vi "SECoP_dataGetAdditionalIndex.vi"(7 "Position":u32, 8 "error in (no error)":errorcluster, 9 "key name":string, 10 "SECoP_dataPtr":T1 {"ptr64" format="%.0x"; "ptr32" format="%.0x"}, 11 "DLL path (in)":T2) -> (0 "error out":errorcluster, 2 "Index":u32, 3 "DLL path (out)":T2)   [LabVIEW 2023, in "SECoP.lvlib"]
doc: "Call <b>\"SECoP_dataGetAdditionalIndex.vi\"</b> to find the index of named additional item of SECoP_dataPtr.\n\n<b>DLL path</b> input and output of cluster from \"SECoP-Initialize.vi\"\n<b>SECoP_dataPtr</b> data to access\n<b>Position</b> points to a virtual flattened entry of the data type\n<b>key name</b> name of the requested additional item of SECoP_dataPtr\n<b>Index</b> index of additional item (or 0xFFFFFFFF if not found)"
uses:
  SECoP.lvlib
  SECoP-libraries.ctl
  SECoP-data.ctl
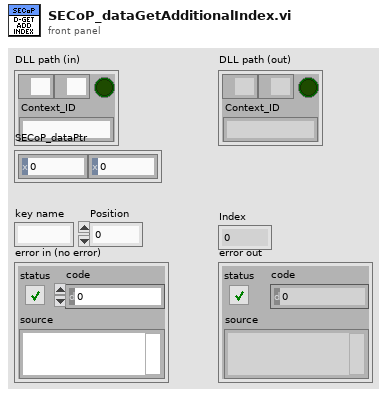
[diagram p1: front panel]
types:
  T1 = typedef "SECoP.lvlib/SECoP-data.ctl" = cluster{"ptr32":u32, "ptr64":u64}
  T2 = typedef "SECoP.lvlib/SECoP-libraries.ctl" = cluster{"serverDLL":path, "variantDLL":path, "cleanup_mode":bool, "Context_ID":string}
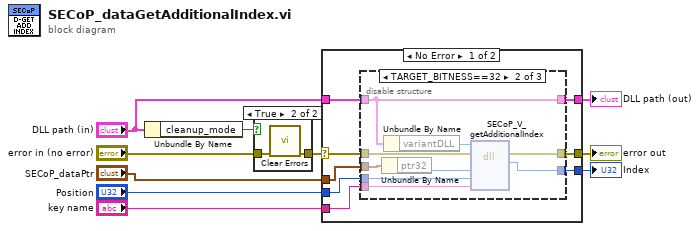
[diagram p0: block diagram]
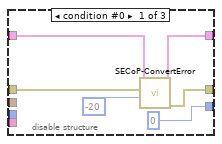
[diagram p3: hidden frame]
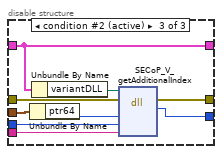
[diagram p4: hidden frame]
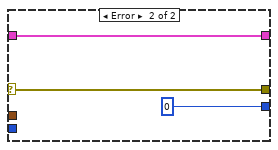
[diagram p5: hidden frame]
diagram:
  n1 = Unbundle By Name("DLL path (in)") -> ("cleanup_mode"=w7:bool)
  n2 = case shown="True" w7 {
    tunnel: "error in (no error)" -> [w11 w13]
    tunnel: [w11 w12] -> w5
    frame False {
    }
    frame True {
      n3 = call <vilib>:"Clear Errors.vi"("error in (no error)"=w13) -> ("error out"=w12:errorcluster)  [unwired: 5 in, 1 out]
    }
  }
  n4 = case shown="No Error" w5 {
    selector: w5 -> [w21 w47]
    tunnel: "DLL path (in)" -> [w20 w48]
    tunnel: [w16 w48] -> w9
    tunnel: [w15 w47] -> w8
    tunnel: "Position" -> [w19 _]
    tunnel: "key name" -> [w18 _]
    tunnel: [w14 u32 0 ("Value")] -> w2
    tunnel: "SECoP_dataPtr" -> [w17 _]
    frame No Error {
      n5 = disable-structure shown="TARGET_BITNESS==32" {
        disable-tunnel: w21 -> [w25 w36 w45]
        disable-tunnel: w20 -> [w27 w28 w38]
        disable-tunnel: [w26 w28 w38] -> w16
        disable-tunnel: [w23 w35 w44] -> w15
        disable-tunnel: w19 -> [_ w34 w43]
        disable-tunnel: w18 -> [_ w33 w42]
        disable-tunnel: [u32 0 ("Index") w30 w39] -> w14
        disable-tunnel: w17 -> [_ w31 w40]
        frame condition #0 {
          n6 = call "SECoP-ConvertError.vi"("return code"=-20, "error in (no error)"=w25, "DLL path (in)"=w27) -> ("error out"=w23:errorcluster, "DLL path (out)"=w26:T2)  [unwired: 7 in]
        }
        frame condition #1 {
          n7 = Unbundle By Name(w31) -> ("ptr32"=w32:u32)
          n8 = Unbundle By Name(w28) -> ("variantDLL"=w29:path)
          n9 = dll-call lib="Z:/Praktische_Aufgaben/SECoP-LabVIEW2015/32bit/SECoP32.dll" fn="SECoP_V_getAdditionalIndex"(path in=w29, error in=w36, "pData"=w32, "uPosition"=w34, "szName"=w33) -> (error out=w35:errorcluster, "return type"=w30:u32)  [unwired: 4 in, 1 out]
        }
        frame condition #2 (active) {
          n10 = Unbundle By Name(w40) -> ("ptr64"=w41:u64)
          n11 = Unbundle By Name(w38) -> ("variantDLL"=w37:path)
          n12 = dll-call lib="Z:/Praktische_Aufgaben/SECoP-LabVIEW2015/32bit/SECoP32.dll" fn="SECoP_V_getAdditionalIndex"(path in=w37, error in=w45, "pData"=w41, "uPosition"=w43, "szName"=w42) -> (error out=w44:errorcluster, "return type"=w39:u32)  [unwired: 4 in, 1 out]
        }
      }
    }
    frame Error {
    }
  }
  "DLL path (out)" <- w9
  "error out" <- w8
  "Index" <- w2
